vi "InstrumentSelection.vi"(8 "error in (no error)":errorcluster, 9 "Verify GPIB address":bool, 10 "Instrument type":T1(ring), 11 "Instrument name IN":string(combo)) -> (0 "error out":errorcluster, 1 "Instrument name OUT":string, 2 "LCR":refnum<class "LCRControl.lvclass">, 3 "Supply":refnum<class "SupplyControl.lvclass">, 4 "Switching":refnum<class "Switching.lvclass">, 5 "Multimeter":refnum<class "MultimeterControl.lvclass">)   [LabVIEW 2013, in "InstrControl.lvclass"]
uses:
  InstrControl.lvclass
  SupplyControl/SupplyControl.lvclass
  LCRControl/LCRControl.lvclass
  MultimeterControl/MultimeterControl.lvclass
  Switching/Switching.lvclass
  SupplyControl/Keithley 2410/KE2410.lvclass
  SupplyControl/Keithley 6517/KE6517.lvclass
  SupplyControl/Keithley 487/KE487.lvclass
  SupplyControl/Keithley 236 & 237/KE236.lvclass
  LCRControl/WK6440B/WK6440B.lvclass
  LCRControl/WK6425/WK6425.lvclass
  LCRControl/HP4263B/HP4263B.lvclass
  MultimeterControl/Keithley 2000/KE2000.lvclass
  Switching/Pickering/Pickering.lvclass
  Switching/Keithley 3706A/KE3706A.lvclass
  InstrumentSetup.vi
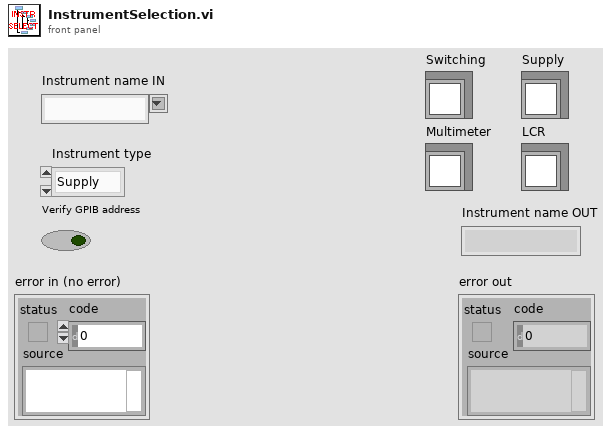
[diagram p1: front panel]
types:
  T1 = enum16{"Supply", "LCR", "Multimeter", "Switching"}
  T2 = cluster{"KE 2410":cluster{"Instrument name":string, "address":refnum<visa-resource-name>, "Instrument type":u16}, "KE 2410_2":cluster{"Instrument name":string, "address":refnum<visa-resource-name>, "Instrument type":u16}, "KE 6517":cluster{"Instrument name":string, "address":refnum<visa-resource-name>, "Instrument type":u16}, "KE 6517_2":cluster{"Instrument name":string, "address":refnum<visa-resource-name>, "Instrument type":u16}, "KE 487":cluster{"Instrument name":string, "address":refnum<visa-resource-name>, "Instrument type":u16}, "KE 236":cluster{"Instrument name":string, "address":refnum<visa-resource-name>, "Instrument type":u16}, "WK 6440B":cluster{"Instrument name":string, "address":refnum<visa-resource-name>, "Instrument type":u16}, "WK 6425":cluster{"Instrument name":string, "address":refnum<visa-resource-name>, "Instrument type":u16}, "HP 4263B":cluster{"Instrument name":string, "address":refnum<visa-resource-name>, "Instrument type":u16}, "Pickering Matrix":cluster{"Instrument name":string, "address":refnum<visa-resource-name>, "Instrument type":u16}, "KE 2000":cluster{"Instrument name":string, "address":refnum<visa-resource-name>, "Instrument type":u16}, "KE3706A Switching":cluster{"Instrument name":string, "address":refnum<visa-resource-name>, "Instrument type":u16}}
  T3 = cluster{"Current Limit":sgl, "Front/Rear Output:":u16, "KE2410":refnum<class "KE2410.lvclass">}
  T4 = cluster{"Current Limit":u16, "Internal meter connect":u16, "KE6517":refnum<class "KE6517.lvclass">}
  T5 = cluster{"Compliance":u16, "Range:":u16, "KE487":refnum<class "KE487.lvclass">}
  T6 = cluster{"current \ncompliance level":dbl, "compliance/\nmeasurement range (auto:0)":u16, "KE236":refnum<class "KE236.lvclass">}
  T7 = cluster{"RC Configuration":u16, "AC amplitude [V]":dbl, "AC frequency [Hz]":i32, "WK6440B":refnum<class "WK6440B.lvclass">}
  T8 = cluster{"RC Configuration":u16, "AC amplitude [V]":dbl, "AC frequency [Hz]":i32, "WK6425":refnum<class "WK6425.lvclass">}
  T9 = cluster{"RC Configuration":u16, "AC amplitude [V]":dbl, "AC frequency [Hz]":i32, "Cable Length":u16, "Averaging":u16, "Averaging Count":i32, "HP4263B":refnum<class "HP4263B.lvclass">}
  T10 = cluster{"Range":u16, "Range Value":dbl, "Function":u16, "KE2000":refnum<class "KE2000.lvclass">}
  T11 = cluster{"Matrix address":string, "Mux1 address":string, "Mux2 address":string, "Pickering":refnum<class "Pickering.lvclass">, "Matrix X Channels":cluster{"Bias Supply / SMU LO":i32, "Bias Supply / SMU HI":i32, "CV Box LO":i32, "CV Box HI":i32, "CV Box LO IN":i32, "CV Box HI IN":i32, "Volt meter LO":i32, "Volt meter HI":i32, "Mux1 C1":i32, "Mux1 C2":i32, "Mux2 C1":i32, "Mux2 C2":i32}}
  T12 = cluster{"Mux1 slot":string, "Mux2 slot":string, "KE3706A":refnum<class "KE3706A.lvclass">}
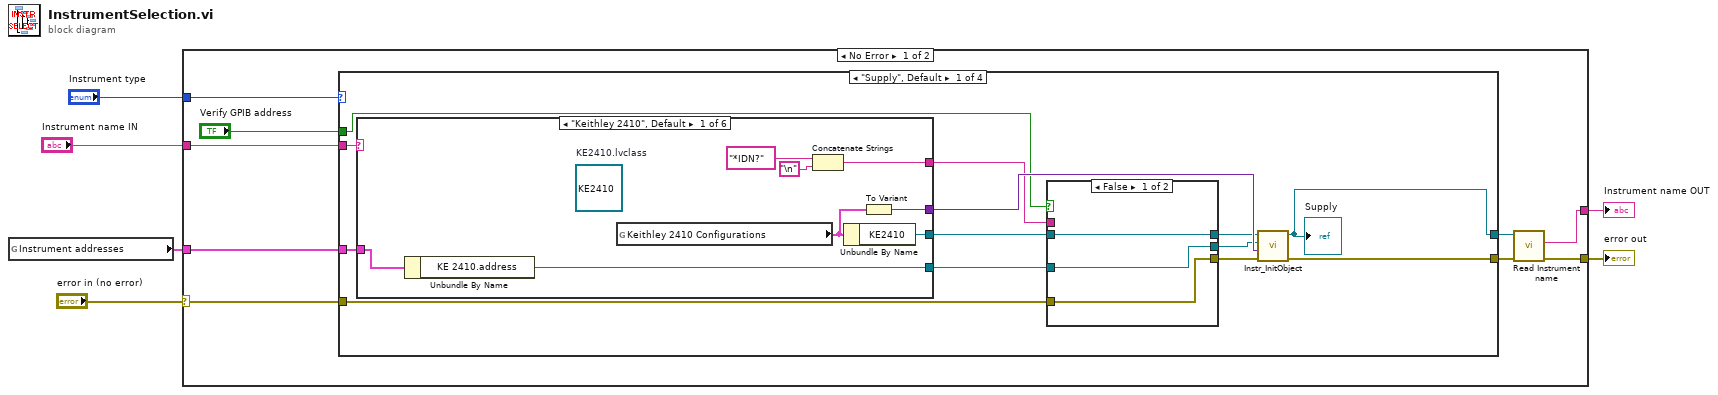
[diagram p0: block diagram]
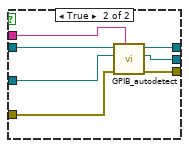
[diagram p2: hidden frame]
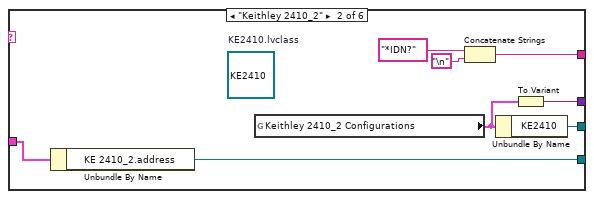
[diagram p3: hidden frame]
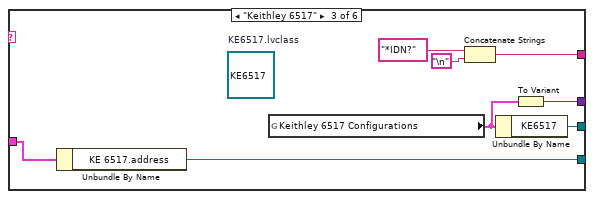
[diagram p4: hidden frame]
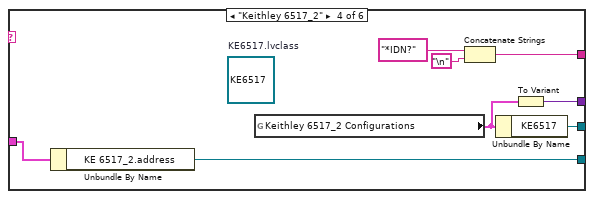
[diagram p5: hidden frame]
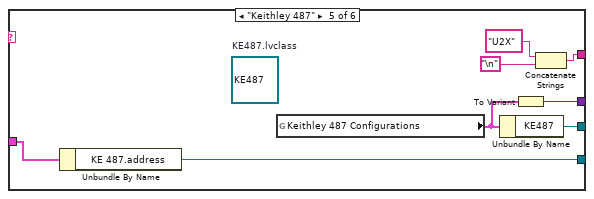
[diagram p6: hidden frame]
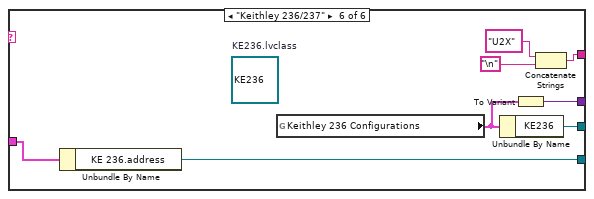
[diagram p7: hidden frame]
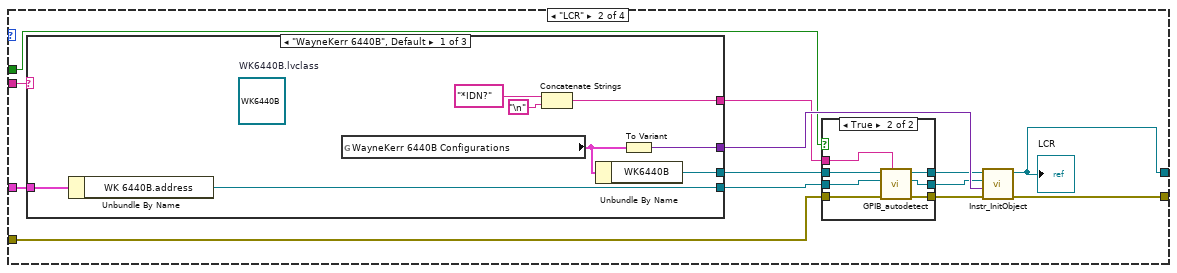
[diagram p8: hidden frame]
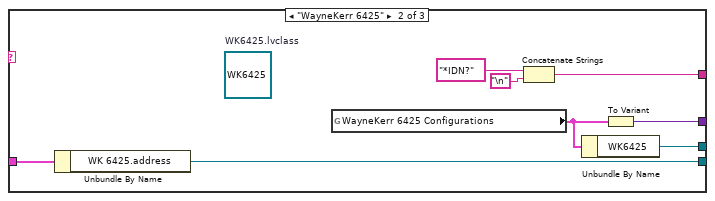
[diagram p10: hidden frame]
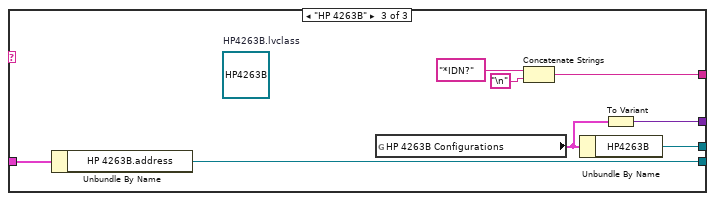
[diagram p11: hidden frame]
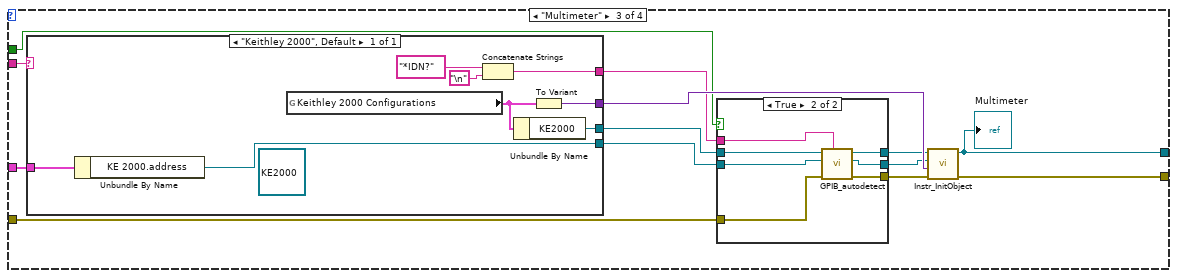
[diagram p12: hidden frame]
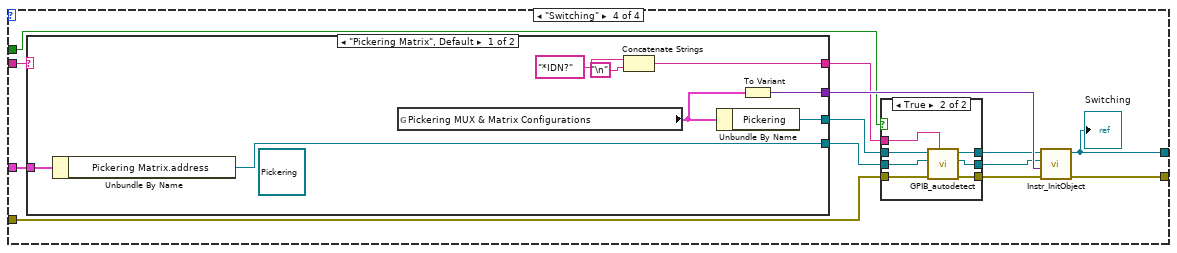
[diagram p14: hidden frame]
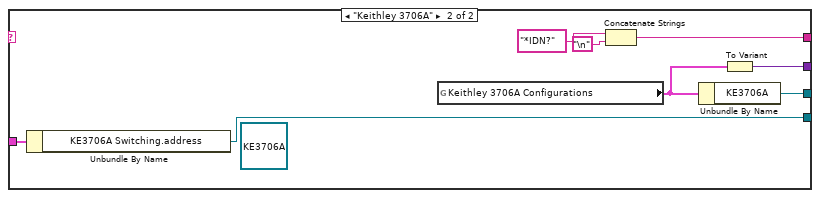
[diagram p16: hidden frame]
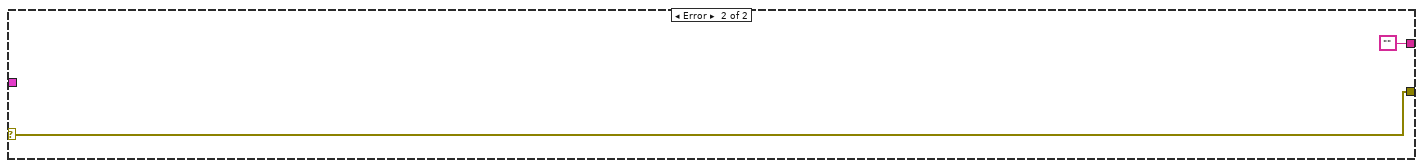
[diagram p17: hidden frame]
diagram:
  n1 = global read "InstrumentSetup.vi" "Instrument addresses"() -> (w1:T2)
  n2 = case shown="No Error" "error in (no error)" {
    selector: "error in (no error)" -> [w13 w205]
    tunnel: [w14 w205] -> w5
    tunnel: [w15 ""] -> w4
    tunnel: "Instrument type" -> [w10 _]
    tunnel: "Instrument name IN" -> [w9 _]
    tunnel: w1 -> [w8 _]
    frame No Error {
      n3 = case shown="\"Supply\", Default" w10 {
        tunnel: w9 -> [w28 w99 w146 w172]
        tunnel: [w27 w97 w144 w176] -> w12
        tunnel: w13 -> [w21 w94 w139 w173]
        tunnel: [w26 w98 w145 w177] -> w11
        tunnel: w8 -> [w25 w96 w143 w175]
        tunnel: "Verify GPIB address" -> [w16 w87 w134 w165]
        frame "Supply", Default {
          n4 = case shown="\"Keithley 2410\", Default" w28 {
            tunnel: [w43 w51 w58 w66 w74 w82] -> w22
            tunnel: w25 -> [w46 w54 w62 w70 w78 w86]
            tunnel: [w45 w53 w61 w69 w77 w85] -> w23
            tunnel: [w44 w52 w60 w68 w76 w84] -> w24
            tunnel: [w39 w47 w55 w63 w71 w79] -> w20
            frame "Keithley 2410", Default {
              (unwired) refnum<class "KE2410.lvclass"> refnum  # KE2410.lvclass
              n5 = Unbundle By Name(w46) -> ("KE 2410.address"=w45:refnum<visa-resource-name>)
              n6 = global read "InstrumentSetup.vi" "Keithley 2410 Configurations"() -> (w42:T3)
              n7 = Concatenate Strings("*IDN?" ("regular expression"), "\n") -> (w39:string)
              n8 = Unbundle By Name(w42) -> ("KE2410"=w43:refnum<class "KE2410.lvclass">)
              n9 = To Variant(anything=w42) -> (Variant=w44:variant)
            }
            frame "Keithley 2410_2" {
              (unwired) refnum<class "KE2410.lvclass"> refnum  # KE2410.lvclass
              n10 = Unbundle By Name(w54) -> ("KE 2410_2.address"=w53:refnum<visa-resource-name>)
              n11 = global read "InstrumentSetup.vi" "Keithley 2410_2 Configurations"() -> (w50:T3)
              n12 = Concatenate Strings("*IDN?" ("regular expression"), "\n") -> (w47:string)
              n13 = Unbundle By Name(w50) -> ("KE2410"=w51:refnum<class "KE2410.lvclass">)
              n14 = To Variant(anything=w50) -> (Variant=w52:variant)
            }
            frame "Keithley 6517" {
              (unwired) refnum<class "KE6517.lvclass"> refnum  # KE6517.lvclass
              n15 = Unbundle By Name(w62) -> ("KE 6517.address"=w61:refnum<visa-resource-name>)
              n16 = global read "InstrumentSetup.vi" "Keithley 6517 Configurations"() -> (w59:T4)
              n17 = Concatenate Strings("*IDN?" ("regular expression"), "\n") -> (w55:string)
              n18 = Unbundle By Name(w59) -> ("KE6517"=w58:refnum<class "KE6517.lvclass">)
              n19 = To Variant(anything=w59) -> (Variant=w60:variant)
            }
            frame "Keithley 6517_2" {
              (unwired) refnum<class "KE6517.lvclass"> refnum  # KE6517.lvclass
              n20 = Unbundle By Name(w70) -> ("KE 6517_2.address"=w69:refnum<visa-resource-name>)
              n21 = global read "InstrumentSetup.vi" "Keithley 6517_2 Configurations"() -> (w67:T4)
              n22 = Concatenate Strings("*IDN?" ("regular expression"), "\n") -> (w63:string)
              n23 = Unbundle By Name(w67) -> ("KE6517"=w66:refnum<class "KE6517.lvclass">)
              n24 = To Variant(anything=w67) -> (Variant=w68:variant)
            }
            frame "Keithley 487" {
              (unwired) refnum<class "KE487.lvclass"> refnum  # KE487.lvclass
              n25 = Unbundle By Name(w78) -> ("KE 487.address"=w77:refnum<visa-resource-name>)
              n26 = global read "InstrumentSetup.vi" "Keithley 487 Configurations"() -> (w75:T5)
              n27 = Unbundle By Name(w75) -> ("KE487"=w74:refnum<class "KE487.lvclass">)
              n28 = To Variant(anything=w75) -> (Variant=w76:variant)
              n29 = Concatenate Strings("U2X" ("regular expression"), "\n") -> (w71:string)
            }
            frame "Keithley 236/237" {
              (unwired) refnum<class "KE236.lvclass"> refnum  # KE236.lvclass
              n30 = Unbundle By Name(w86) -> ("KE 236.address"=w85:refnum<visa-resource-name>)
              n31 = global read "InstrumentSetup.vi" "Keithley 236 Configurations"() -> (w83:T6)
              n32 = Unbundle By Name(w83) -> ("KE236"=w82:refnum<class "KE236.lvclass">)
              n33 = To Variant(anything=w83) -> (Variant=w84:variant)
              n34 = Concatenate Strings("U2X" ("regular expression"), "\n") -> (w79:string)
            }
          }
          n35 = case shown="False" w16 {
            tunnel: w23 -> [w30 w38]
            tunnel: w22 -> [w31 w37]
            tunnel: w21 -> [w29 w36]
            tunnel: w20 -> [_ w35]
            tunnel: [w30 w34] -> w19
            tunnel: [w31 w33] -> w18
            tunnel: [w29 w32] -> w17
            frame False {
            }
            frame True {
              n36 = call-dynamic "GPIB_autodetect.vi"("ID command"=w35, "error in (no error)"=w36, "Instrument address in"=w38, "InstrControl in"=w37) -> ("error out"=w32:errorcluster, "Instrument address out"=w34:refnum<visa-resource-name>, "InstrControl out"=w33:refnum<class "SupplyControl.lvclass">)  [unwired: 5 in]
            }
          }
          n37 = call-dynamic "Instr_InitObject.vi"("error in (no error)"=w17, "Instrument Configuration"=w24, "Instrument address"=w19, "SupplyControl in"=w18) -> ("error out"=w26:errorcluster, "SupplyControl out"=w27:refnum<class "SupplyControl.lvclass">)  [unwired: 6 in]
          "Supply" <- w27
        }
        frame "LCR" {
          n38 = case shown="\"WayneKerr 6440B\", Default" w99 {
            tunnel: [w113 w121 w128] -> w92
            tunnel: w96 -> [w117 w125 w130]
            tunnel: [w116 w124 w129] -> w93
            tunnel: [w115 w123 w126] -> w95
            tunnel: [w110 w118 w131] -> w91
            frame "WayneKerr 6440B", Default {
              (unwired) refnum<class "WK6440B.lvclass"> refnum  # WK6440B.lvclass
              n39 = Unbundle By Name(w117) -> ("WK 6440B.address"=w116:refnum<visa-resource-name>)
              n40 = global read "InstrumentSetup.vi" "WayneKerr 6440B Configurations"() -> (w114:T7)
              n41 = Concatenate Strings("*IDN?" ("regular expression"), "\n") -> (w110:string)
              n42 = Unbundle By Name(w114) -> ("WK6440B"=w113:refnum<class "WK6440B.lvclass">)
              n43 = To Variant(anything=w114) -> (Variant=w115:variant)
            }
            frame "WayneKerr 6425" {
              (unwired) refnum<class "WK6425.lvclass"> refnum  # WK6425.lvclass
              n44 = Unbundle By Name(w125) -> ("WK 6425.address"=w124:refnum<visa-resource-name>)
              n45 = global read "InstrumentSetup.vi" "WayneKerr 6425 Configurations"() -> (w122:T8)
              n46 = Concatenate Strings("*IDN?" ("regular expression"), "\n") -> (w118:string)
              n47 = Unbundle By Name(w122) -> ("WK6425"=w121:refnum<class "WK6425.lvclass">)
              n48 = To Variant(anything=w122) -> (Variant=w123:variant)
            }
            frame "HP 4263B" {
              (unwired) refnum<class "HP4263B.lvclass"> refnum  # HP4263B.lvclass
              n49 = Unbundle By Name(w130) -> ("HP 4263B.address"=w129:refnum<visa-resource-name>)
              n50 = global read "InstrumentSetup.vi" "HP 4263B Configurations"() -> (w127:T9)
              n51 = Concatenate Strings("*IDN?" ("regular expression"), "\n") -> (w131:string)
              n52 = Unbundle By Name(w127) -> ("HP4263B"=w128:refnum<class "HP4263B.lvclass">)
              n53 = To Variant(anything=w127) -> (Variant=w126:variant)
            }
          }
          n54 = case shown="True" w87 {
            tunnel: w94 -> [w100 w109]
            tunnel: w93 -> [w102 w108]
            tunnel: w92 -> [w101 w107]
            tunnel: w91 -> [_ w106]
            tunnel: [w100 w105] -> w90
            tunnel: [w102 w104] -> w89
            tunnel: [w101 w103] -> w88
            frame False {
            }
            frame True {
              n55 = call-dynamic "GPIB_autodetect.vi"("ID command"=w106, "error in (no error)"=w109, "Instrument address in"=w108, "InstrControl in"=w107) -> ("error out"=w105:errorcluster, "Instrument address out"=w104:refnum<visa-resource-name>, "InstrControl out"=w103:refnum<class "LCRControl.lvclass">)  [unwired: 5 in]
            }
          }
          n56 = call-dynamic "Instr_InitObject.vi"("error in (no error)"=w90, "Instrument Configuration"=w95, "Instrument address"=w89, "LCRControl in"=w88) -> ("error out"=w98:errorcluster, "LCRControl out"=w97:refnum<class "LCRControl.lvclass">)  [unwired: 6 in]
          "LCR" <- w97
        }
        frame "Multimeter" {
          n57 = case shown="\"Keithley 2000\", Default" w146 {
            tunnel: [w160] -> w140
            tunnel: w143 -> [w164]
            tunnel: [w163] -> w141
            tunnel: [w162] -> w142
            tunnel: [w157] -> w138
            frame "Keithley 2000", Default {
              (unwired) refnum<class "KE2000.lvclass"> refnum ("KE2000.lvclass")
              n58 = Unbundle By Name(w164) -> ("KE 2000.address"=w163:refnum<visa-resource-name>)
              n59 = global read "InstrumentSetup.vi" "Keithley 2000 Configurations"() -> (w161:T10)
              n60 = Concatenate Strings("*IDN?" ("regular expression"), "\n") -> (w157:string)
              n61 = Unbundle By Name(w161) -> ("KE2000"=w160:refnum<class "KE2000.lvclass">)
              n62 = To Variant(anything=w161) -> (Variant=w162:variant)
            }
          }
          n63 = case shown="True" w134 {
            tunnel: w141 -> [w147 w156]
            tunnel: w140 -> [w149 w155]
            tunnel: w139 -> [w148 w154]
            tunnel: w138 -> [_ w153]
            tunnel: [w147 w152] -> w137
            tunnel: [w149 w151] -> w136
            tunnel: [w148 w150] -> w135
            frame False {
            }
            frame True {
              n64 = call-dynamic "GPIB_autodetect.vi"("ID command"=w153, "error in (no error)"=w154, "Instrument address in"=w156, "InstrControl in"=w155) -> ("error out"=w150:errorcluster, "Instrument address out"=w152:refnum<visa-resource-name>, "InstrControl out"=w151:refnum<class "KE2000.lvclass">)  [unwired: 5 in]
            }
          }
          n65 = call-dynamic "Instr_InitObject.vi"("error in (no error)"=w135, "Instrument Configuration"=w142, "Instrument address"=w137, "KE2000 in"=w136) -> ("error out"=w145:errorcluster, "KE2000 out"=w144:refnum<class "KE2000.lvclass">)  [unwired: 6 in]
          "Multimeter" <- w144
        }
        frame "Switching" {
          n66 = case shown="\"Pickering Matrix\", Default" w172 {
            tunnel: w175 -> [w195 w200]
            tunnel: [w194 w199] -> w174
            tunnel: [w192 w197] -> w171
            tunnel: [w191 w201] -> w170
            tunnel: [w188 w198] -> w169
            frame "Pickering Matrix", Default {
              (unwired) refnum<class "Pickering.lvclass"> refnum ("Pickering")
              n67 = Unbundle By Name(w195) -> ("Pickering Matrix.address"=w194:refnum<visa-resource-name>)
              n68 = global read "InstrumentSetup.vi" "Pickering MUX & Matrix Configurations"() -> (w193:T11)
              n69 = Concatenate Strings("*IDN?" ("regular expression"), "\n") -> (w188:string)
              n70 = Unbundle By Name(w193) -> ("Pickering"=w191:refnum<class "Pickering.lvclass">)
              n71 = To Variant(anything=w193) -> (Variant=w192:variant)
            }
            frame "Keithley 3706A" {
              (unwired) refnum<class "KE3706A.lvclass"> refnum ("KE3700A in")
              n72 = Unbundle By Name(w200) -> ("KE3706A Switching.address"=w199:refnum<visa-resource-name>)
              n73 = global read "InstrumentSetup.vi" "Keithley 3706A Configurations"() -> (w203:T12)
              n74 = Concatenate Strings("*IDN?" ("regular expression"), "\n") -> (w198:string)
              n75 = Unbundle By Name(w203) -> ("KE3706A"=w201:refnum<class "KE3706A.lvclass">)
              n76 = To Variant(anything=w203) -> (Variant=w197:variant)
            }
          }
          n77 = case shown="True" w165 {
            tunnel: w174 -> [w179 w187]
            tunnel: w173 -> [w180 w186]
            tunnel: w170 -> [w178 w185]
            tunnel: w169 -> [_ w184]
            tunnel: [w178 w183] -> w168
            tunnel: [w180 w182] -> w167
            tunnel: [w179 w181] -> w166
            frame False {
            }
            frame True {
              n78 = call-dynamic "GPIB_autodetect.vi"("ID command"=w184, "error in (no error)"=w186, "Instrument address in"=w187, "InstrControl in"=w185) -> ("error out"=w182:errorcluster, "Instrument address out"=w181:refnum<visa-resource-name>, "InstrControl out"=w183:refnum<class "Switching.lvclass">)  [unwired: 5 in]
            }
          }
          n79 = call-dynamic "Instr_InitObject.vi"("error in (no error)"=w167, "Instrument Configuration"=w171, "Instrument address"=w166, "Switching in"=w168) -> ("error out"=w177:errorcluster, "Switching out"=w176:refnum<class "Switching.lvclass">)  [unwired: 6 in]
          "Switching" <- w176
        }
      }
      n80 = call-dynamic "Read Instrument name.vi"("error in (no error)"=w11, "InstControl in"=w12) -> ("error out"=w14:errorcluster, "Instrument name"=w15:string)  [unwired: 7 in, 1 out]
    }
    frame Error {
    }
  }
  "error out" <- w5
  "Instrument name OUT" <- w4
